vi "Write Name.vi"(8 "error in (no error)":errorcluster, 10 "Name":string, 11 "_Shared in":refnum<class "_Shared.lvclass">) -> (0 "error out":errorcluster, 3 "_Shared out":refnum<class "_Shared.lvclass">)   [LabVIEW 2021, in "_Rename.lvlib" / "_Shared.lvclass"]
uses:
  _Shared.lvclass
  _Shared.lvclass/_Shared.ctl
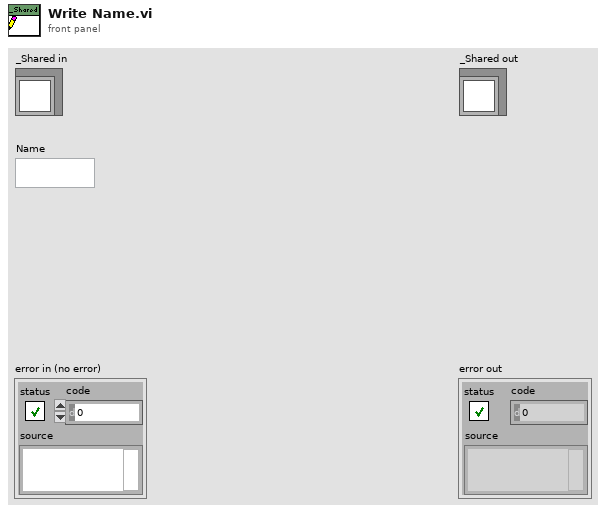
[diagram p1: front panel]
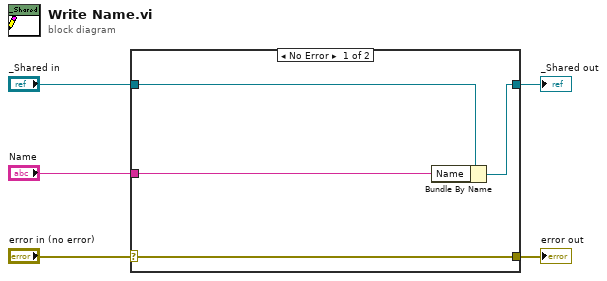
[diagram p0: block diagram]
diagram:
  n1 = case shown="No Error" "error in (no error)" {
    selector: "error in (no error)" -> [w9 w10]
    tunnel: [w9 w10] -> w4
    tunnel: [w7 w11] -> w2
    tunnel: "_Shared in" -> [w8 w11]
    tunnel: "Name" -> [w6 _]
    frame No Error {
      n2 = Bundle By Name(cluster=w8, "Name"=w6) -> (w7:refnum<class "_Shared.lvclass">)
    }
    frame Error {
    }
  }
  "error out" <- w4
  "_Shared out" <- w2
